vi "to string array.vi"(8 "error in (no error)":errorcluster, 11 "PID Module configuration in":refnum<class "PID Module configuration.lvclass">) -> (0 "error out":errorcluster, 1 "Array":string[][](array[string]), 2 "version":string, 3 "PID Module configuration out":refnum<class "PID Module configuration.lvclass">)   [LabVIEW 2015, in "PID Module configuration.lvclass"]
uses:
  PID Module configuration.lvclass
  PID Module configuration.lvclass/PID Module configuration.ctl
  Read Lines.vi
  <vilib>/NI/Tag Bus/tag/default value polymorphs/read default value Double.vi
  <vilib>/NI/Tag Bus Module Framework/channel/TBM channel.lvclass
  <vilib>/NI/Tag Bus/tag/tag descriptor.lvclass
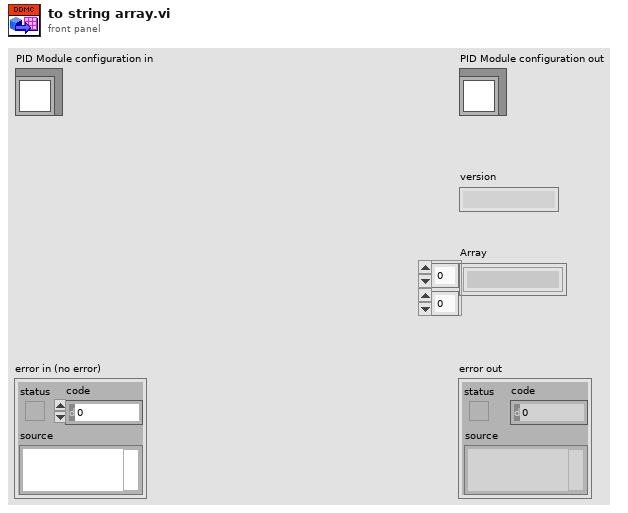
[diagram p1: front panel]
types:
  T1 = typedef "PID Module 2 configuration.lvclass/Line.ctl" = cluster{"PID ID":string, "Setpoint":refnum<class "TBM channel.lvclass">, "Variable":refnum<class "TBM channel.lvclass">, "Output":refnum<class "TBM channel.lvclass">, "Output High":refnum<class "TBM channel.lvclass">, "Output Low":refnum<class "TBM channel.lvclass">, "P":refnum<class "TBM channel.lvclass">, "I":refnum<class "TBM channel.lvclass">, "D":refnum<class "TBM channel.lvclass">}
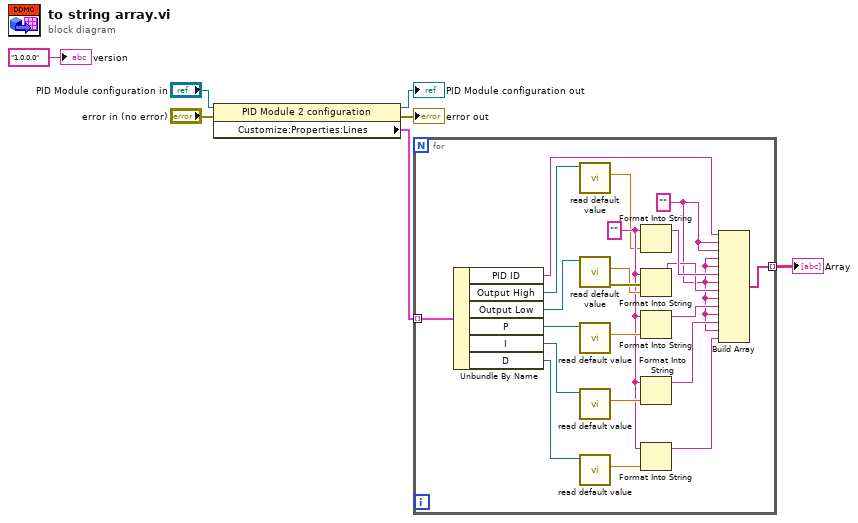
[diagram p0: block diagram]
diagram:
  n1 = property class="PID Module 2 configuration"(reference="PID Module configuration in", error in="error in (no error)") -> (reference out=→"PID Module configuration out":refnum<class "PID Module configuration.lvclass">, error out=→"error out":errorcluster, "Customize:Properties:Lines"=w4:T1[])
  n2 = for {
    tunnel: w4 -> [w28] mode=indexing
    tunnel: [w27] -> w1 mode=indexing
    w15 = "" ("initial string")
    w8 = "" ("element")
    n3 = Unbundle By Name(w28) -> ("PID ID"=w26:string, "Output High"=w25:refnum<class "TBM channel.lvclass">, "Output Low"=w24:refnum<class "TBM channel.lvclass">, "P"=w23:refnum<class "TBM channel.lvclass">, "I"=w22:refnum<class "TBM channel.lvclass">, "D"=w21:refnum<class "TBM channel.lvclass">)
    n4 = call-poly <vilib>:"read default value.vi"("system tag in"=w25) -> ("default value"=w13:dbl)  [unwired: 7 in, 3 out]
    n5 = call-poly <vilib>:"read default value.vi"("system tag in"=w24) -> ("error out"=w20:errorcluster, "default value"=w16:dbl)  [unwired: 7 in, 2 out]
    n6 = call-poly <vilib>:"read default value.vi"("system tag in"=w23) -> ("default value"=w17:dbl)  [unwired: 7 in, 3 out]
    n7 = call-poly <vilib>:"read default value.vi"("system tag in"=w22) -> ("default value"=w18:dbl)  [unwired: 7 in, 3 out]
    n8 = call-poly <vilib>:"read default value.vi"("system tag in"=w21) -> ("default value"=w19:dbl)  [unwired: 7 in, 3 out]
    n9 = Format Into String(initial string=w15, w13) -> (resulting string=w14:string)  [unwired: 2 in, 1 out]
    n10 = Format Into String(initial string=w15, error in=w20, w16) -> (resulting string=w12:string)  [unwired: 1 in, 1 out]
    n11 = Format Into String(initial string=w15, w17) -> (resulting string=w11:string)  [unwired: 2 in, 1 out]
    n12 = Format Into String(initial string=w15, w18) -> (resulting string=w10:string)  [unwired: 2 in, 1 out]
    n13 = Format Into String(initial string=w15, w19) -> (resulting string=w9:string)  [unwired: 2 in, 1 out]
    n14 = Build Array(w26, w8, w8, w8, w8, w14, w8, w12, w8, w11, w8, w10, w8, w9) -> (w27:string[])
  }
  "Array" <- w1
  "version" <- "1.0.0.0" ("version")
